vi "Get Start Tag.vi"(8 "error in (no error)":errorcluster, 11 "Element in":refnum<class "Element.lvclass">) -> (0 "error out":errorcluster, 2 "Start Tag":string, 3 "Element out":refnum<class "Element.lvclass">)   [LabVIEW 2026, in "VILab.lvlib" / "Element.lvclass"]
uses:
  Element.lvclass
  <vilib>/AdvancedString/1D String Array to Delimited String (string).vi
  Element.lvclass/Element.ctl
  VILab.lvlib
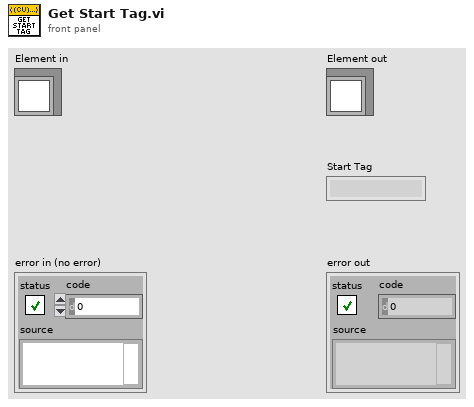
[diagram p1: front panel]
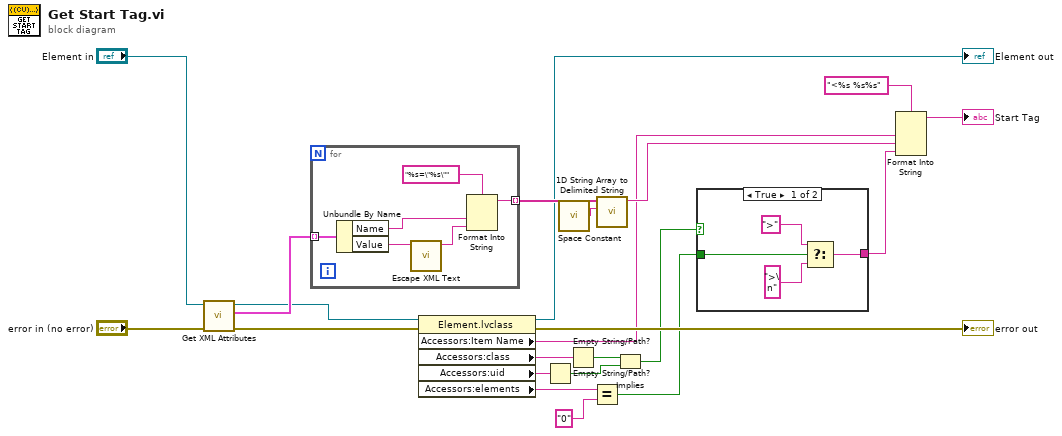
[diagram p0: block diagram]
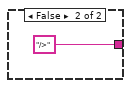
[diagram p2: hidden frame]
diagram:
  n1 = call-dynamic "Get XML Attributes.vi"("error in (no error)"="error in (no error)", "Element in"="Element in") -> ("error out"=w21:errorcluster, "XML Attributes"=w18:cluster{"Name":string, "Value":string}[], "Element out"=w8:refnum<class "Element.lvclass">)  [unwired: 7 in]
  n2 = for {
    tunnel: w18 -> [w28] mode=indexing
    tunnel: [w23] -> w14 mode=indexing
    n3 = Unbundle By Name(w28) -> ("Name"=w24:string, "Value"=w27:string)
    n4 = call "Escape XML Text.vi"("String"=w27) -> ("Escaped String"=w25:string)  [unwired: 10 in]
    n5 = Format Into String(format string="%s=\"%s\"", w24, w25) -> (resulting string=w23:string)  [unwired: 2 in, 1 out]
  }
  n6 = property class="Element.lvclass"(reference=w8, error in=w21) -> (reference out=→"Element out":refnum<class "Element.lvclass">, error out=→"error out":errorcluster, "Accessors:Item Name"=w4:string, "Accessors:class"=w5:string, "Accessors:uid"=w12:string, "Accessors:elements"=w3:string)
  n7 = Empty String/Path?(string/path=w12) -> (empty?=w10:bool)
  n8 = call <vilib>:"Space Constant.vi"() -> ("String"=w16:string)
  n9 = Empty String/Path?(string/path=w5) -> (empty?=w11:bool)
  n10 = Equal?(x=w3, y="0") -> (x = y?=w1:bool)
  n11 = call-poly <vilib>:"1D String Array to Delimited String.vi"("delimiter"=w16, "string array"=w14) -> ("delimited string"=w15:string)  [unwired: 9 in]
  n12 = Implies(1:w10, 2:w11) -> (0:w9:bool)
  n13 = case shown="True" w9 {
    tunnel: [w30 "/>"] -> w6
    tunnel: w1 -> [w29 _]
    frame True {
      n14 = Select(t=">", s=w29, f=">\n") -> (s? t:f=w30:string)
    }
    frame False {
    }
  }
  n15 = Format Into String(format string="<%s %s%s", w4, w15, w6) -> (resulting string=→"Start Tag":string)  [unwired: 2 in, 1 out]
